vi "workbook add chart.vi"(8 "error in (no error)":errorcluster, 10 "chart_type":T1 items=["LXW_CHART_NONE", "LXW_CHART_AREA", "LXW_CHART_AREA_STACKED", "LXW_CHART_AREA_STACKED_PERCENT", "LXW_CHART_BAR", "LXW_CHART_BAR_STACKED", "LXW_CHART_BAR_STACKED_PERCENT", "LXW_CHART_COLUMN", "LXW_CHART_COLUMN_STACKED", "LXW_CHART_COLUMN_STACKED_PERCENT", "LXW_CHART_DOUGHNUT", "LXW_CHART_LINE", "LXW_CHART_LINE_STACKED", "LXW_CHART_LINE_STACKED_PERCENT", "LXW_CHART_PIE", "LXW_CHART_SCATTER", "LXW_CHART_SCATTER_STRAIGHT", "LXW_CHART_SCATTER_STRAIGHT_WITH_MARKERS", "LXW_CHART_SCATTER_SMOOTH", "LXW_CHART_SCATTER_SMOOTH_WITH_MARKERS", "LXW_CHART_RADAR", "LXW_CHART_RADAR_WITH_MARKERS", "LXW_CHART_RADAR_FILLED", "LXW_CHART_STOCK"], 11 "workbook":u32) -> (0 "error out":errorcluster, 3 "function return":u32)   [LabVIEW 8.6]
doc: "lxw_chart workbook_add_chart(lxw_workbook workbook, uint8_t chart_type);"
uses:
  pending_lvxlsxwriter/xlsxwriter.dll
  Controls/lxw_chart_type.ctl
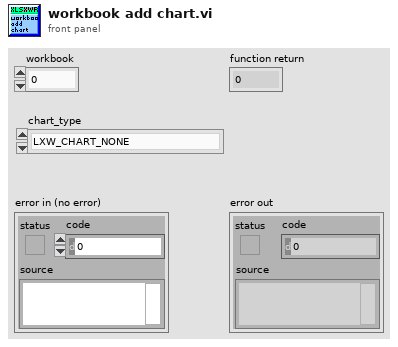
[diagram p1: front panel]
types:
  T1 = typedef "lxw_chart_type.ctl" = u8
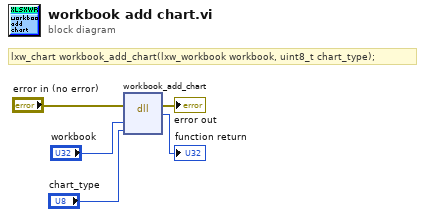
[diagram p0: block diagram]
diagram:
  # "lxw_chart workbook_add_chart(lxw_workbook workbook, uint8_t chart_type);"
  n1 = dll-call lib="C:/Users/WDAGUtilityAccount/Desktop/pending_lvxlsxwriter/xlsxwriter.*" fn="workbook_add_chart"(error in="error in (no error)", "workbook"="workbook", "chart_type"="chart_type") -> (error out=→"error out":errorcluster, →"function return":u32)  [unwired: 4 in, 1 out]
